vi "Lookup Channel.vi"(8 "error in (no error)":errorcluster, 11 "ChannelService in":refnum<class "ChannelService.lvclass">) -> (0 "error out":errorcluster, 3 "ChannelService out":refnum<class "ChannelService.lvclass">)   [LabVIEW 2024, in "Vecto.lvlib" / "ChannelService.lvclass"]
uses:
  ChannelService.lvclass
  ChannelService.lvclass/ChannelService.ctl
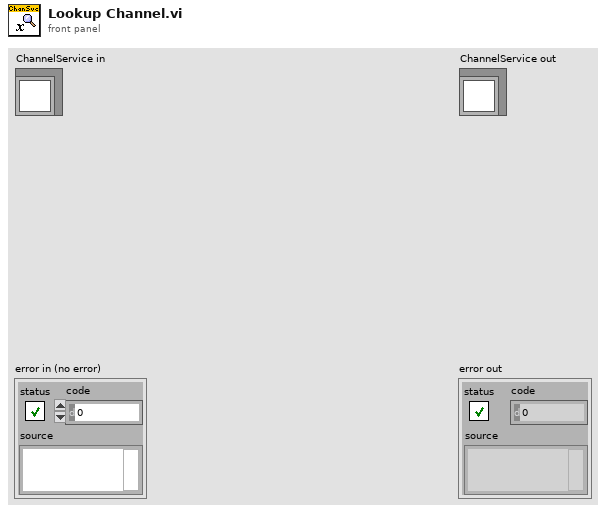
[diagram p1: front panel]
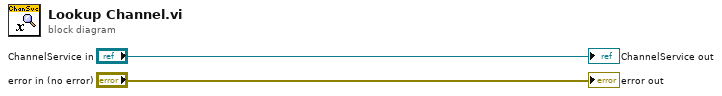
[diagram p0: block diagram]
diagram:
  "error out" <- "error in (no error)"
  "ChannelService out" <- "ChannelService in"
